vi "Noise (G3) - Defaults.vi"() -> (3 "persistent":T1={"Show Aweight"=TRUE})   [LabVIEW 2020, in "Noise (G3).xctl"]
uses:
  Noise (G3).xctl
  Noise (G3) - Persistent.ctl
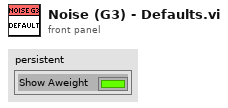
[diagram p1: front panel]
types:
  T1 = typedef "Noise (G3).xctl/Noise (G3) - Persistent.ctl" = cluster{"Show Aweight":bool}
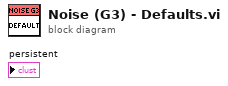
[diagram p0: block diagram]
diagram:
